vi "Configure Level.vi"   [LabVIEW 2018, in "Agilent MXA Series.lvlib"]
doc: "Configures the vertical settings of the spectrum analyzer."
uses:
  Agilent MXA Series.lvlib
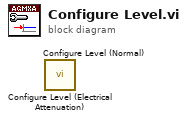
[diagram p0: block diagram]
diagram:
  n1 = call "Configure Level (Electrical Attenuation).vi"() -> ()  [unwired: 14 in, 2 out]
  n2 = call "Configure Level (Normal).vi"() -> ()  [unwired: 14 in, 2 out]
